vi "To Probe.vi"(8 "error in (no error)":errorcluster, 11 "Is Probeable in":refnum<class "Is Probeable.lvclass">) -> (0 "error out":errorcluster, 2 "Probe":T1, 3 "Is Probeable out":refnum<class "Is Probeable.lvclass">)   [LabVIEW 2020, in "PV Access.lvlib" / "PV Data.lvlib" / "Is Probeable.lvclass"]
uses:
  Is Probeable.lvclass
  Has Time Stamp/Has Time Stamp.lvclass
  Has Alarm/Has Alarm.lvclass
  Probe.ctl
  PV Data.lvlib
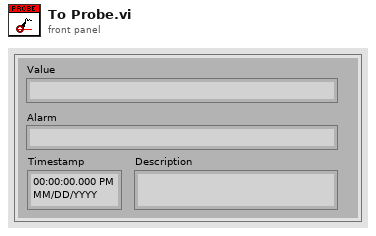
[diagram p1: front panel]
types:
  T1 = typedef "PV Access.lvlib/PV Data.lvlib/Probe.ctl" = cluster{"Timestamp":timestamp, "Value":string, "Description":string, "Alarm":string}
  T2 = typedef "PV Access.lvlib/PV Data.lvlib/Alarm.ctl" = cluster{"Severity":T3, "Status":T4, "Message":string}
  T3 = typedef "PV Access.lvlib/PV Data.lvlib/Alarm Severity.ctl" = enum32{"no", "minor", "major", "record", "invalid", "undefined"}
  T4 = typedef "PV Access.lvlib/PV Data.lvlib/Alarm Status.ctl" = enum32{"no", "device", "driver", "record", "db", "conf", "undefined", "client"}
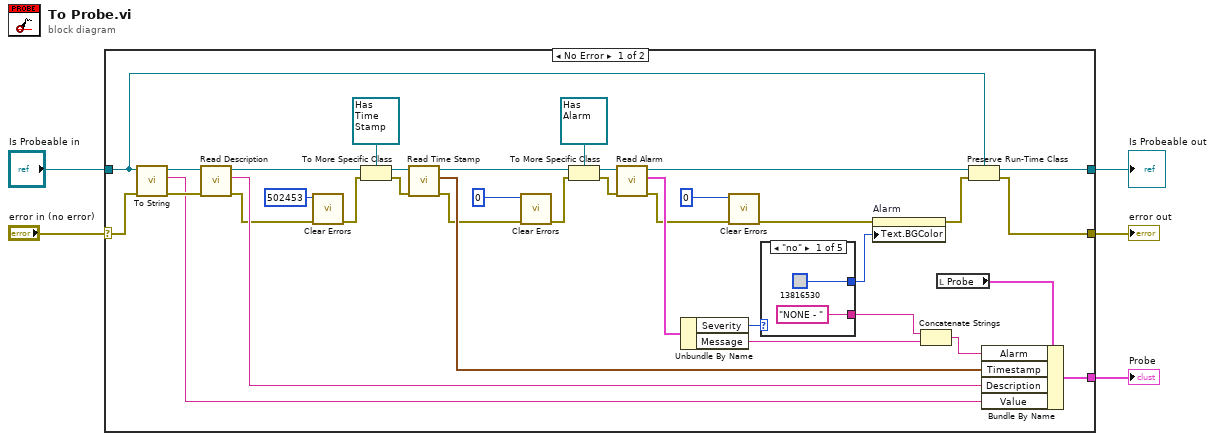
[diagram p0: block diagram]
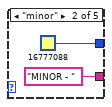
[diagram p2: hidden frame]
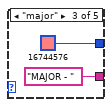
[diagram p3: hidden frame]
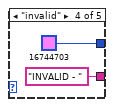
[diagram p4: hidden frame]
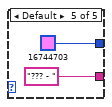
[diagram p5: hidden frame]
diagram:
  n1 = case shown="No Error" "error in (no error)" {
    selector: "error in (no error)" -> [w39 w53]
    tunnel: [w6 w53] -> w3
    tunnel: "Is Probeable in" -> [w9 w52]
    tunnel: [w41 _] -> w1
    tunnel: [w11 w52] -> w2
    frame No Error {
      n2 = call-dynamic "To String.vi"("error in (no error)"=w39, "Is Stringifiable in"=w9) -> ("error out"=w26:errorcluster, "string"=w23:string, "Is Stringifiable out"=w25:refnum<class "Is Probeable.lvclass">)  [unwired: 7 in]
      n3 = call-dynamic "Read Description.vi"("error in (no error)"=w26, "Base Interface in"=w25) -> ("error out"=w19:errorcluster, "description"=w22:string, "Base Interface out"=w24:refnum<class "Is Probeable.lvclass">)  [unwired: 7 in]
      n4 = call <vilib>:"Clear Errors.vi"("error in (no error)"=w19, "specific error code to clear (0: all)"=502453) -> ("error out"=w18:errorcluster)  [unwired: 4 in, 1 out]
      n5 = To More Specific Class(target class=refnum<class "Has Time Stamp.lvclass"> refnum ("PV Access.lvlib:PV Data.lvlib:Has Time Stamp.lvclass"), reference=w24, error in=w18) -> (specific class reference=w33:refnum<class "Has Time Stamp.lvclass">, error out=w34:errorcluster)
      n6 = call-dynamic "Read Time Stamp.vi"("error in"=w34, "Has Timestamp in"=w33) -> ("error out"=w16:errorcluster, "time stamp"=w21:timestamp, "Has Timestamp out"=w14:refnum<class "Has Time Stamp.lvclass">)  [unwired: 6 in, 1 out]
      n7 = call <vilib>:"Clear Errors.vi"("error in (no error)"=w16, "specific error code to clear (0: all)"=0) -> ("error out"=w15:errorcluster)  [unwired: 4 in, 1 out]
      n8 = To More Specific Class(target class=refnum<class "Has Alarm.lvclass"> refnum ("PV Access.lvlib:PV Data.lvlib:Has Alarm.lvclass"), reference=w14, error in=w15) -> (specific class reference=w31:refnum<class "Has Alarm.lvclass">, error out=w30:errorcluster)
      n9 = call-dynamic "Read Alarm.vi"("error in"=w30, "Has Alarm in"=w31) -> ("error out"=w12:errorcluster, "alarm"=w29:T2, "Has Alarm out"=w10:refnum<class "Has Alarm.lvclass">)  [unwired: 7 in]
      n10 = Unbundle By Name(w29) -> ("Severity"=w28:T3, "Message"=w27:string)
      n11 = call <vilib>:"Clear Errors.vi"("error in (no error)"=w12, "specific error code to clear (0: all)"=0) -> ("error out"=w8:errorcluster)  [unwired: 4 in, 1 out]
      n12 = case shown="\"no\"" w28 {
        tunnel: [u32 13816530 ("Text.BGColor") u32 16777088 ("Text.BGColor") u32 16744576 ("Text.BGColor") u32 16744703 ("Text.BGColor") u32 16744703 ("Text.BGColor")] -> w36
        tunnel: ["NONE - " "MINOR - " "MAJOR - " "INVALID - " "??? - "] -> w38
        frame "no" {
        }
        frame "minor" {
        }
        frame "major" {
        }
        frame "invalid" {
        }
        frame Default {
        }
      }
      n13 = property on="Alarm" class="Str"(error in=w8, "Text.BGColor"=w36) -> (error out=w7:errorcluster)  [unwired: 1 in, 1 out]
      n14 = Concatenate Strings(w38, w27) -> (w37:string)
      n15 = local read "Probe"() -> (w40:T1)
      n16 = Preserve Run-Time Class(object in=w10, error in=w7, 2:w9) -> (object out=w11:refnum<class "Is Probeable.lvclass">, error out=w6:errorcluster)
      n17 = Bundle By Name(cluster=w40, "Alarm"=w37, "Timestamp"=w21, "Description"=w22, "Value"=w23) -> (w41:T1)
    }
    frame Error {
    }
  }
  "error out" <- w3
  "Is Probeable out" <- w2
  "Probe" <- w1
